vi "kalmanRobot.vi"(0 "robots_yellow in":T1[](array[typedef]) {"height" format="%+4.3f"; "pixel_y" format="%+4.3f"; "pixel_x" format="%+4.3f"; "orientation" format="%+4.3f"; "y" format="%+4.3f"; "confidence" format="%4.3f"; "x" format="%+4.3f"}, 3 "Time Stamp 2":timestamp=timestamp(3583818425.330139 s since 1904-01-01), 5 "error in (no error)":errorcluster) -> (14 "robots_yellow out":T1[](array[typedef]) {"height" format="%+4.3f"; "pixel_y" format="%+4.3f"; "pixel_x" format="%+4.3f"; "orientation" format="%+4.3f"; "y" format="%+4.3f"; "confidence" format="%4.3f"; "x" format="%+4.3f"}, 19 "error out":errorcluster)   [LabVIEW 2023, in "Vision.lvclass"]
uses:
  Vision.lvclass
  Old vision/Controls/SSL Detection Robot.ctl
  <vilib>/Analysis/Matrix/Datatypes/RealMatrix.ctl
  <vilib>/Analysis/coordinate.llb/Wrap Angle (scalar).vi
  <vilib>/Analysis/Matrix/Numeric/Conversions/Array To Matrix - RA.vi
  <vilib>/Analysis/Matrix/NI_Matrix.lvlib
  <vilib>/Analysis/NI_AAL_Angle.lvlib
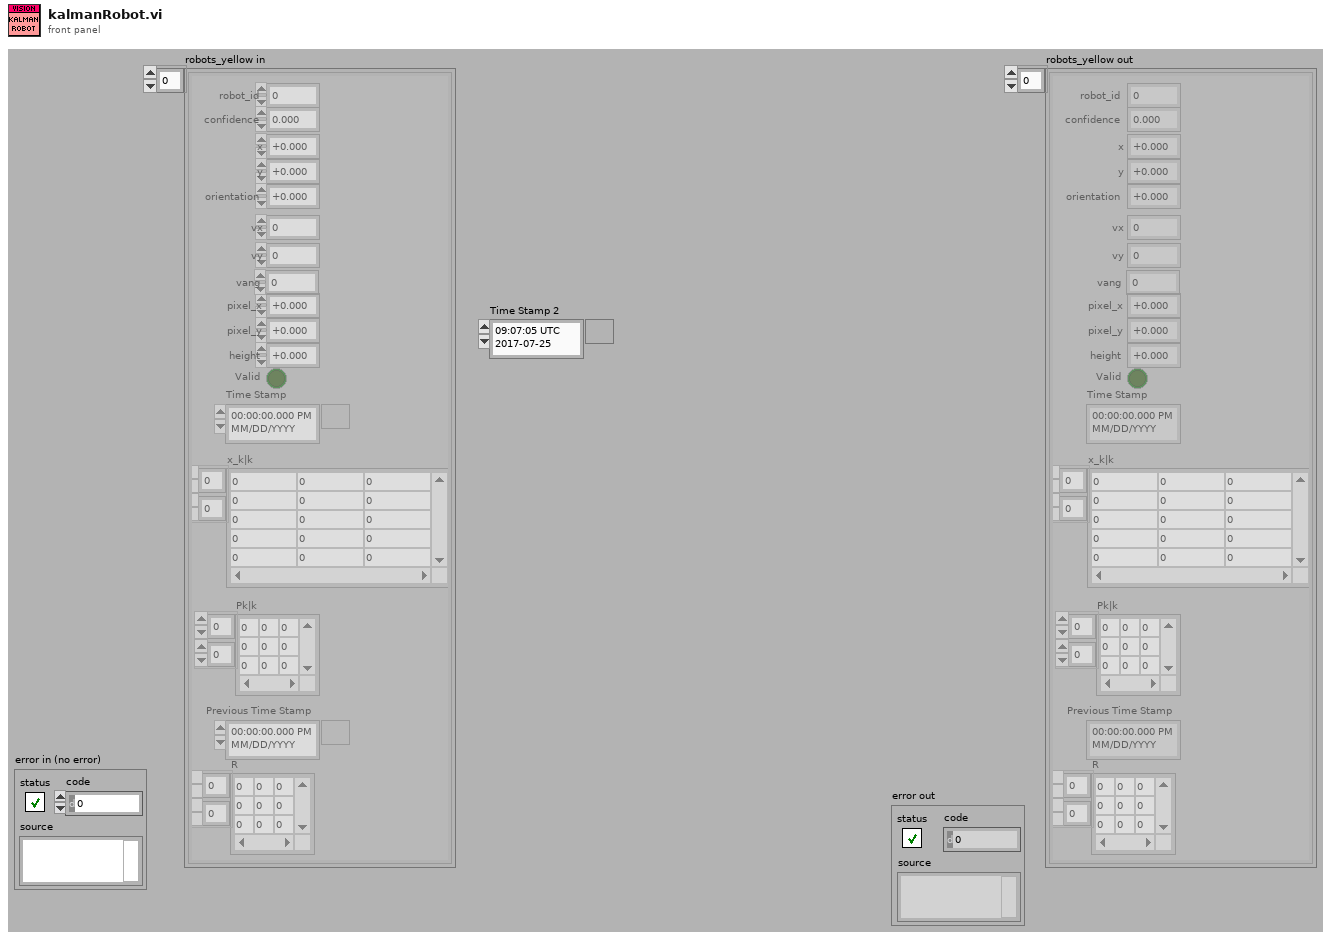
[diagram p1: front panel]
types:
  T1 = typedef "SSL Detection Robot.ctl" = cluster{"x":sgl, "robot_id":u32, "confidence":sgl, "y":sgl, "orientation":sgl, "pixel_x":sgl, "pixel_y":sgl, "height":sgl, "Valid":bool, "Time Stamp":timestamp, "x_k|k":T2, "Pk|k":T2, "Previous Time Stamp":timestamp, "R":T2, "vx":dbl, "vy":dbl, "vang":dbl}
  T2 = typedef "NI_Matrix.lvlib/RealMatrix.ctl" = dbl[][]
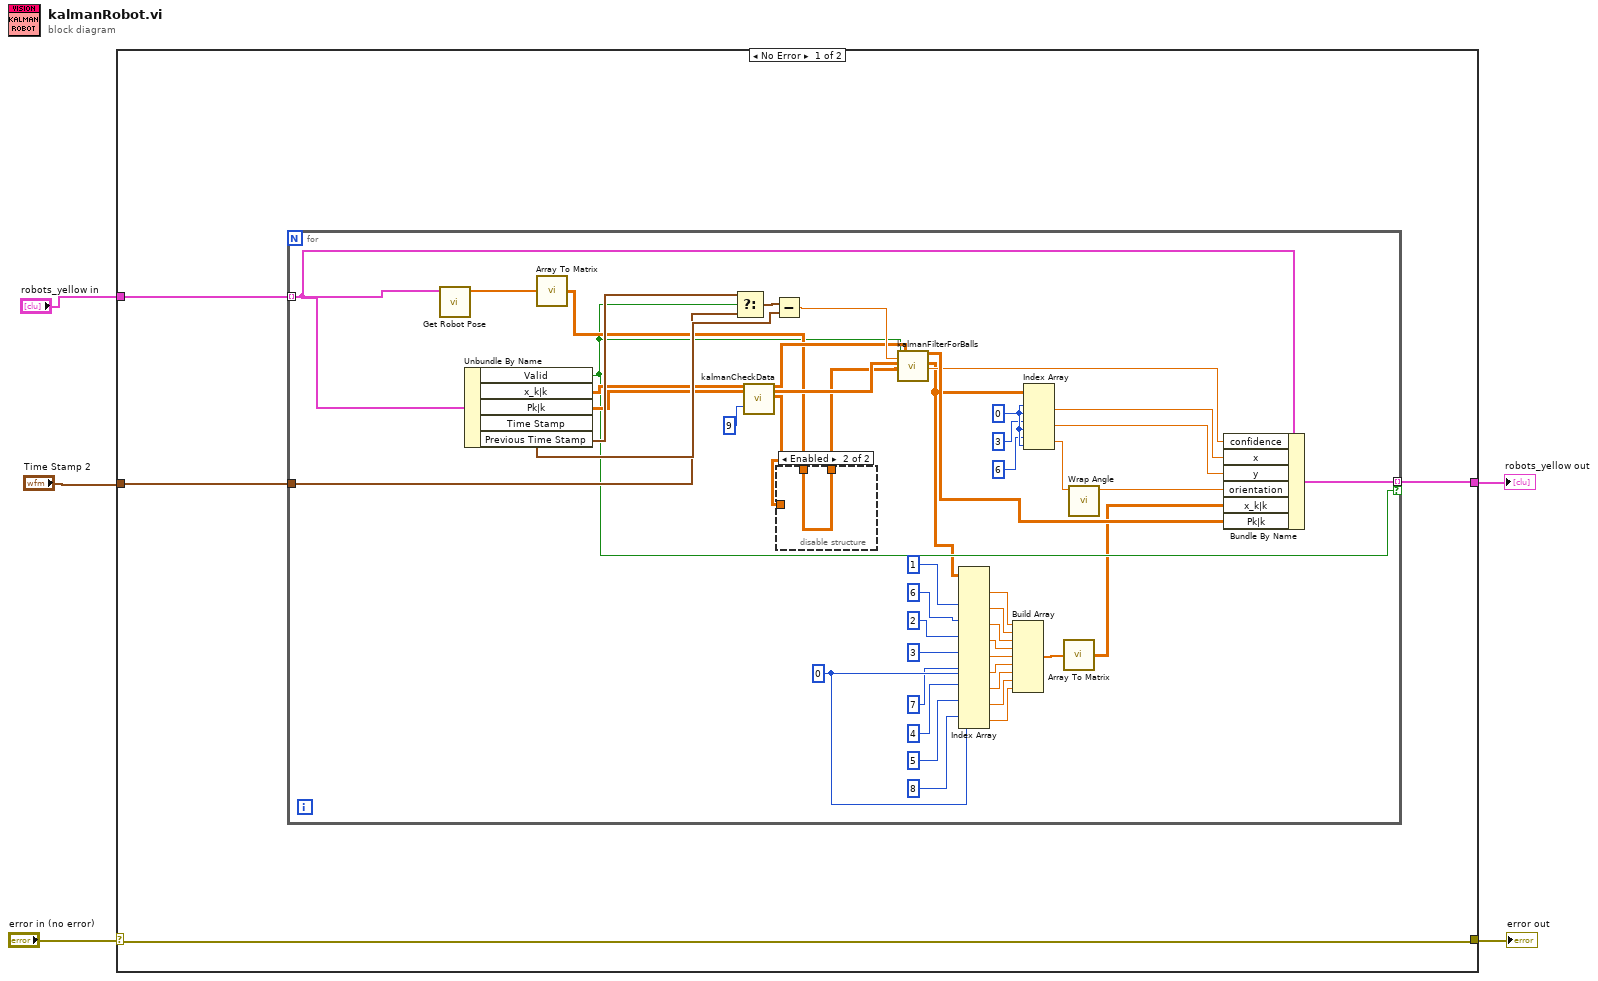
[diagram p0: block diagram]
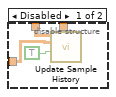
[diagram p2: hidden frame]
diagram:
  n1 = case shown="No Error" "error in (no error)" {
    selector: "error in (no error)" -> [w9 w62]
    tunnel: [w9 w62] -> w4
    tunnel: "Time Stamp 2" -> [w8 _]
    tunnel: "robots_yellow in" -> [w7 _]
    tunnel: [w6 _] -> w1
    frame No Error {
      n2 = for {
        tunnel: w7 -> [w38] mode=indexing
        tunnel: [w49] -> w6 mode=indexing if=w33
        tunnel: w8 -> [w54]
        w29 = 0
        w52 = 0 ("index (row)")
        n3 = call "Get Robot Pose.vi"("Detection Robot"=w38) -> ("Pose"=w37:sgl[])  [unwired: 10 in]
        n4 = Unbundle By Name(w38) -> ("Valid"=w33:bool, "x_k|k"=w42:T2, "Pk|k"=w43:T2, "Time Stamp"=w55:timestamp, "Previous Time Stamp"=w56:timestamp)
        n5 = call-poly <vilib>:"Array To Matrix.vi"("Real 1D Array"=w37) -> ("Real Matrix (Column Vector)"=w36:T2)
        n6 = Select(t=w55, s=w33, f=w54) -> (s? t:f=w53:timestamp)
        n7 = call "kalmanCheckData.vi"("x_k"=w42, "Pk"=w43, "Variance Memory"=9) -> ("x_k out"=w41:T2, "Pk out"=w39:T2, "R out"=w40:T2)  [unwired: 13 in, 1 out]
        n8 = Subtract(x=w53, y=w56) -> (x-y=w48:dbl)
        n9 = disable-structure shown="Enabled" {
          disable-tunnel: [w59 w61] -> w32
          disable-tunnel: w36 -> [w58 w61]
          disable-tunnel: w40 -> [w57 _]
          frame Disabled {
            n10 = call "Update Sample History.vi"("Ball?"=TRUE, "R in"=w57, "Sample"=w58) -> ("Sample Unwrapped"=w59:T2)  [unwired: 6 in, 2 out]
          }
          frame Enabled {
          }
        }
        n11 = call "kalmanFilterForBalls.vi"("Use Observation"=w33, "intervalo"=w48, "Pk-1|k-1"=w39, "z_k"=w32, "x_k-1|k-1"=w41) -> ("Pk|k out"=w47:T2, "x_k|k out"=w30:T2, "Conf"=w46:dbl)  [unwired: 11 in, 1 out]
        n12 = Index Array(array=w30, index (row) #1=w29, index (col) #1=w29, index (row) #2=1 ("disabled index (row)"), index (col) #2=w29, index (row) #3=6 ("disabled index (row)"), index (col) #3=w29, index (row) #4=2 ("disabled index (row)"), index (col) #4=w29, index (row) #5=3 ("index (col)"), index (col) #5=w29, index (row) #6=7 ("index (col)"), index (col) #6=w29, index (row) #7=4 ("disabled index (row)"), index (col) #7=w29, index (row) #8=5 ("disabled index (row)"), index (col) #8=w29, index (row) #9=8 ("disabled index (row)"), index (col) #9=w29) -> (element #1=w20:dbl, element #2=w19:dbl, element #3=w18:dbl, element #4=w17:dbl, element #5=w16:dbl, element #6=w15:dbl, element #7=w14:dbl, element #8=w13:dbl, element #9=w12:dbl)
        n13 = Build Array(w20, w19, w18, w17, w16, w15, w14, w13, w12) -> (w11:dbl[])
        n14 = Index Array(array=w30, index (row) #1=w52, index (col) #1=w52, index (row) #2=3 ("disabled index (col)"), index (col) #2=w52, index (row) #3=6 ("disabled index (col)"), index (col) #3=w52) -> (element #1=w31:dbl, element #2=w45:dbl, element #3=w34:dbl)
        n15 = call-poly <vilib>:"Array To Matrix.vi"("Real 1D Array"=w11) -> ("Real Matrix (Column Vector)"=w10:T2)
        n16 = call-poly <vilib>:"Wrap Angle.vi"("angle in"=w34) -> ("angle out"=w35:dbl)  [unwired: 9 in, 1 out]
        n17 = Bundle By Name(cluster=w38, "confidence"=w46, "x"=w31, "y"=w45, "orientation"=w35, "x_k|k"=w10, "Pk|k"=w47) -> (w49:T1)
      }
    }
    frame Error {
    }
  }
  "error out" <- w4
  "robots_yellow out" <- w1
